vi "SE5082_Configure_system.vi"(8 "error in":errorcluster, 11 "VISA resource name in":refnum<visa-resource-name>="USB0::0x168C::0x5082::0000217419::INSTR") -> (0 "error out":errorcluster={"status"=TRUE, "code"=-1073807305, "source"="VISA Read in SE5082_Configure_system.vi->test_GUI_with_seq.vi"}, 3 "VISA resource name out":refnum<visa-resource-name>="USB0::0x168C::0x5082::0000217419::INSTR")   [LabVIEW 2017]
panel:
  in  "Readout status?":bool
  in  "Read-out commands":string[](array[string])=[":ROSC:SOUR?", ":ROSC:EXT:FREQ?", ":INST:COUP:STATE?"]
  out "Input waveform commands":string[](array[string])=[":SOUR:ROSC:SOUR EXT", ":SOUR:ROSC:EXT:FREQ 10M", ":INST:COUP:STATE ON"]
  out "Status output":string[](array[string])=["EXT\n", "10M\n", "ON\n", "", "", ""]
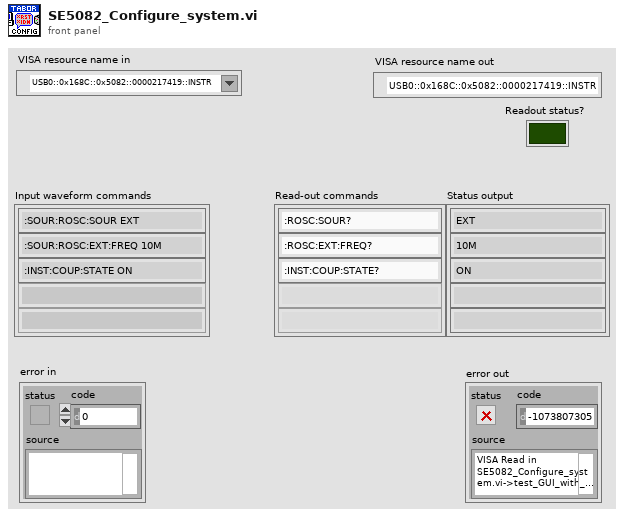
[diagram p1: front panel]
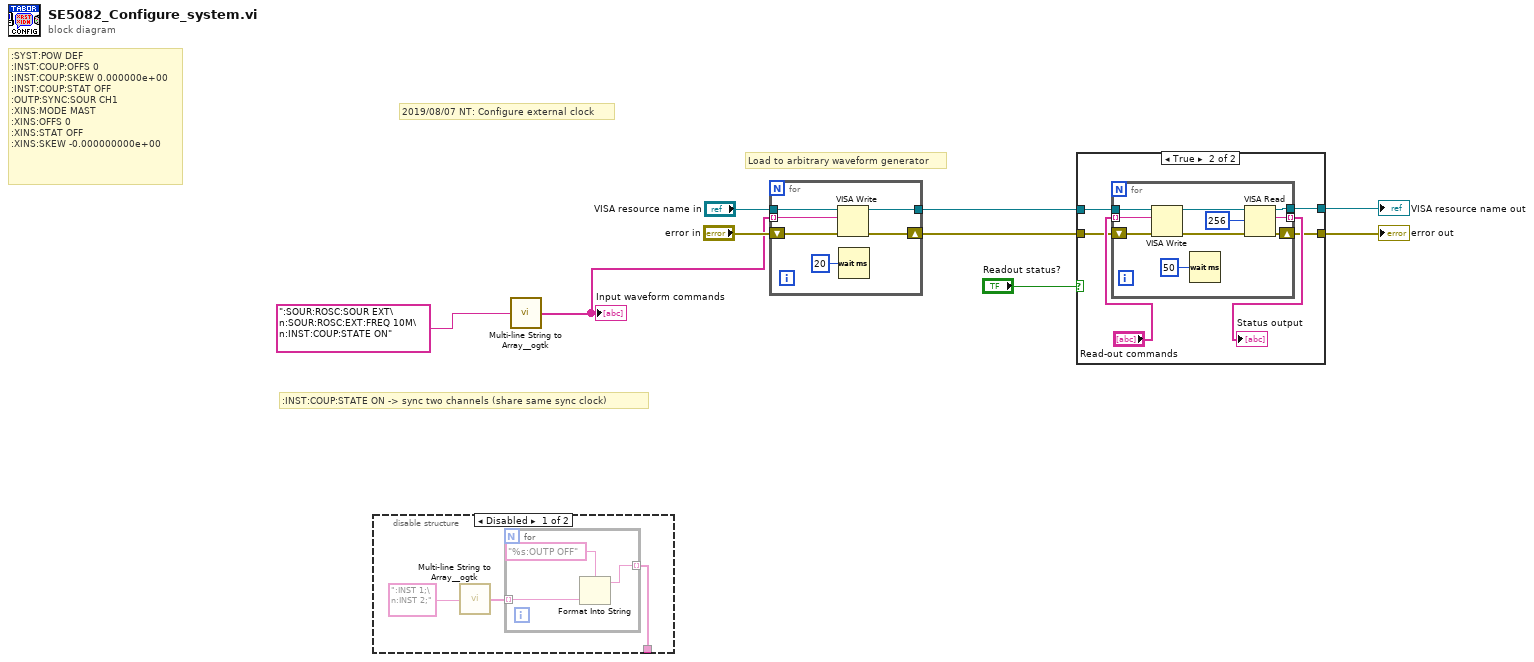
[diagram p0: block diagram]
diagram:
  # ":INST:COUP:STATE ON -> sync two channels (share same sync clock)"
  # ":SYST:POW DEF\n:INST:COUP:OFFS 0\n:INST:COUP:SKEW 0.000000e+00\n:INST:COUP:STAT OFF\n:OUTP:SYNC:SOUR CH1\n:XINS:MODE MAST\n:XINS:OFFS 0\n:XINS:STAT OFF\n:XINS:SKEW -0.000000000e+00"
  # "2019/08/07 NT: Configure external clock"
  # "Load to arbitrary waveform generator"
  n1 = disable-structure shown="Disabled" {
    disable-tunnel: [w10 _] -> _
    frame Disabled {
      n2 = call <userlib>:"Multi-line String to Array__ogtk.vi"("string"=":INST 1;\n:INST 2;" ("initial string")) -> ("lines"=w11:string[])
      n3 = for {
        tunnel: w11 -> [w13] mode=indexing
        tunnel: [w14] -> w10 mode=indexing
        n4 = Format Into String(format string="%s:OUTP OFF", w13) -> (resulting string=w14:string)  [unwired: 2 in, 1 out]
      }
    }
    frame Enabled {
    }
  }
  n5 = call <userlib>:"Multi-line String to Array__ogtk.vi"("string"=":SOUR:ROSC:SOUR EXT\n:SOUR:ROSC:EXT:FREQ 10M\n:INST:COUP:STATE ON" ("write buffer")) -> ("lines"=w1:string[])
  "Input waveform commands" <- w1
  n6 = for {
    tunnel: "VISA resource name in" -> [w21]
    tunnel: w1 -> [w16] mode=indexing
    shift-right: [w19] -> w7
    shift-left: "error in" -> [w20]
    tunnel: [w18] -> w8
    n7 = VISA Write(VISA resource name=w21, write buffer=w16, error in (no error)=w20) -> (VISA resource name out=w18:refnum<visa-resource-name>, error out=w19:errorcluster)  [unwired: 1 out]
    n8 = Wait (ms)(milliseconds to wait=u32 20) -> ()  [unwired: 1 out]
  }
  n9 = case shown="True" "Readout status?" {
    tunnel: w8 -> [w23 w27]
    tunnel: w7 -> [w22 w26]
    tunnel: [w22 w25] -> w6
    tunnel: [w23 w24] -> w5
    frame False {
    }
    frame True {
      n10 = for {
        tunnel: [w36] -> w29 mode=indexing
        shift-right: [w35] -> w25
        shift-left: w26 -> [w32]
        tunnel: w27 -> [w34]
        tunnel: "Read-out commands" -> [w33] mode=indexing
        tunnel: [w30] -> w24
        n11 = VISA Write(VISA resource name=w34, write buffer=w33, error in (no error)=w32) -> (VISA resource name out=w38:refnum<visa-resource-name>, error out=w37:errorcluster)  [unwired: 1 out]
        n12 = Wait (ms)(milliseconds to wait=u32 50) -> ()  [unwired: 1 out]
        n13 = VISA Read(VISA resource name=w38, byte count=u32 256, error in (no error)=w37) -> (VISA resource name out=w30:refnum<visa-resource-name>, read buffer=w36:string, error out=w35:errorcluster)  [unwired: 1 out]
      }
      "Status output" <- w29
    }
  }
  "error out" <- w6
  "VISA resource name out" <- w5
